vi "Start Heartbeat Checker.vi"(8 "Error In":errorcluster, 10 "Interval":i32, 11 "reference in":refnum<class "Network Mangement.lvclass">) -> (0 "Error Out":errorcluster, 3 "reference out":refnum<class "Network Mangement.lvclass">)   [LabVIEW 2024, in "CANopen Master.lvlib" / "Network Mangement.lvclass"]
uses:
  Network Mangement.lvclass
  Heartbeat Checker.vi
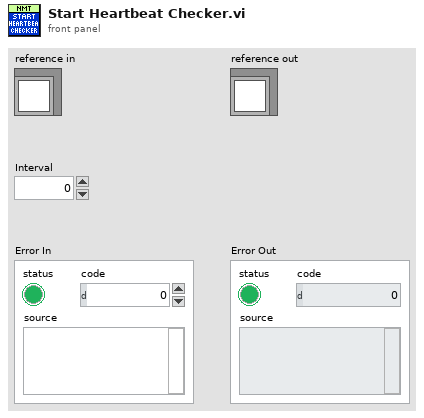
[diagram p1: front panel]
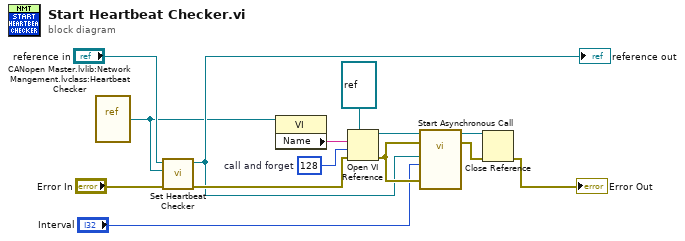
[diagram p0: block diagram]
diagram:
  w13 = 128  # call and forget
  n1 = vi-ref "CANopen Master.lvlib:Network Mangement.lvclass:Heartbeat Checker.vi"() -> (w2:refnum<vi>)
  n2 = call "Set Heartbeat Checker.vi"("Error In"="Error In", "Heartbeat Checker"=w2, "reference in"="reference in") -> ("Error Out"=w5:errorcluster, "reference out"=w3:refnum<class "Network Mangement.lvclass">)  [unwired: 7 in]
  "reference out" <- w3
  n3 = property class="VI"(reference=w2) -> ("Name"=w8:string)  [unwired: 1 in, 2 out]
  n4 = Open VI Reference(type specifier VI Refnum (for type only)=refnum<vi> refnum, vi path=w8, options=w13, error in (no error)=w5) -> (vi reference=w12:refnum<vi>, error out=w9:errorcluster)  [unwired: 2 in]
  n5 = call-by-ref "Start Asynchronous Call"(reference=w12, error in=w9, "Error In"=w9, "Interval"="Interval", "reference in"=w3) -> (reference out=w11:refnum<vi>, error out=w10:errorcluster)  [unwired: 9 in]
  n6 = Close Reference(reference=w11, error in (no error)=w10) -> (error out=→"Error Out":errorcluster)
